vi "Draw Attitude Indicator.vi"(5 "FcdVI Refnum":refnum<vi>, 7 "2D Picture":refnum<vi>, 9 "State in":T1={"Draw Options"={"Text Color"=16777238, "Wing Color"=16751616, "Dial Outline Color"=13816530, "Sky Color"=3381759, "Ground Color"=8213043, "Horizon Line Color"=16777225, "Outline Color"=0, "Dial Background Color"=5987163, "Draw Wings"=TRUE, "Draw Text"=TRUE, "Font Name"="Helvetica", "Angle units"=enum."Degrees"}}, 10 "Data in":T4) -> (3 "Picture Out":picture)   [LabVIEW 2017, in "Attitude Indicator.xctl"]
uses:
  <vilib>/robotics/Controls/Attitude Indicator/Attitude Indicator.xctl
  <vilib>/robotics/Controls/Attitude Indicator/_Attitude Indicator Support Files/Attitude Indicator Data.ctl
  <vilib>/robotics/Controls/Attitude Indicator/_Attitude Indicator Support Files/Attitude Indicator State.ctl
  <vilib>/robotics/Controls/Attitude Indicator/Attitude Picture/Draw Options.ctl
  <vilib>/robotics/Controls/Utilities/Angle Units.ctl
  <vilib>/Utility/miscctls.llb/LVBoundsTypeDef.ctl
  <vilib>/Utility/miscctls.llb/LVPositionTypeDef.ctl
  <vilib>/robotics/Controls/Attitude Indicator/Attitude Picture/NI_Robotics_Attitude Picture.lvlib
  <vilib>/robotics/Controls/Utilities/NI_Robotics_Control Utilities.lvlib
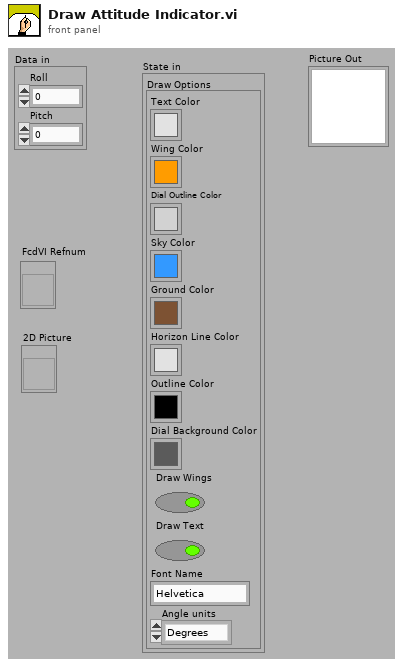
[diagram p1: front panel]
types:
  T1 = typedef "Attitude Indicator.xctl/Attitude Indicator State.ctl" = cluster{"Draw Options":T2}
  T2 = typedef "NI_Robotics_Attitude Picture.lvlib/Draw Options.ctl" = cluster{"Text Color":u32, "Wing Color":u32, "Dial Outline Color":u32, "Sky Color":u32, "Ground Color":u32, "Horizon Line Color":u32, "Outline Color":u32, "Dial Background Color":u32, "Draw Wings":bool, "Draw Text":bool, "Font Name":string, "Angle units":T3}
  T3 = typedef "NI_Robotics_Control Utilities.lvlib/Angle Units.ctl" = enum16{"Radians", "Degrees"}
  T4 = typedef "Attitude Indicator.xctl/Attitude Indicator Data.ctl" = cluster{"Roll":dbl, "Pitch":dbl}
  T5 = typedef "LVPositionTypeDef.ctl" = cluster{"Left":i32, "Top":i32}
  T6 = typedef "LVBoundsTypeDef.ctl" = cluster{"Width":u32, "Height":u32}
  T7 = typedef "LVRectTypeDef.ctl" = cluster{"Left":i16, "Top":i16, "Right":i16, "Bottom":i16}
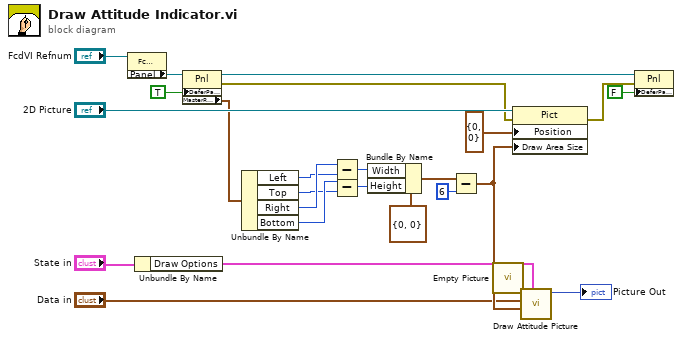
[diagram p0: block diagram]
diagram:
  n1 = property class="FcdVI"(reference="FcdVI Refnum") -> ("Panel"=w23:refnum<vi>)  [unwired: 1 in, 2 out]
  n2 = Unbundle By Name("State in") -> ("Draw Options"=w4:T2)
  n3 = property class="Pnl"(reference=w23, "DeferPanUpdts"=TRUE ("Defer Panel Updates")) -> (reference out=w21:refnum<vi>, error out=w19:errorcluster, "MasterRect"=w17:T7)  [unwired: 1 in]
  n4 = Unbundle By Name(w17) -> ("Left"=w15:i16, "Top"=w13:i16, "Right"=w16:i16, "Bottom"=w14:i16)
  n5 = Subtract(x=w16, y=w15) -> (x-y=w11:i16)
  n6 = Subtract(x=w14, y=w13) -> (x-y=w10:i16)
  n7 = Bundle By Name(cluster=T6 {"Width"=0, "Height"=0} ("Draw Area Size"), "Width"=w11, "Height"=w10) -> (w9:T6)
  n8 = Subtract(x=w9, y=u32 6) -> (x-y=w3:T6)
  n9 = call "Empty Picture"() -> ("empty picture"=w1:picture)
  n10 = property class="Pict"(reference="2D Picture", error in=w19, "Position"=T5 {"Left"=0, "Top"=0}, "Draw Area Size"=w3) -> (error out=w18:errorcluster)  [unwired: 1 out]
  n11 = call <vilib>:"Draw Attitude Picture.vi"("draw options"=w4, "DrawAreaSize"=w3, "attitude"="Data in", "picture in"=w1) -> ("picture out"=→"Picture Out":picture)  [unwired: 6 in, 1 out]
  n12 = property class="Pnl"(reference=w21, error in=w18, "DeferPanUpdts"=FALSE ("Defer Panel Updates")) -> ()  [unwired: 2 out]
